vi "File_NewPathGeneartor.vi"(0 "NewPath":path, 1 "OldPath":path, 2 "NewName":string, 3 "OldName":string, 4 "NewSuffix":string, 5 "OldSuffix":string) -> (14 "PathOut":path, 16 "NameOut":string, 18 "SuffixOut":string)   [LabVIEW 2020]
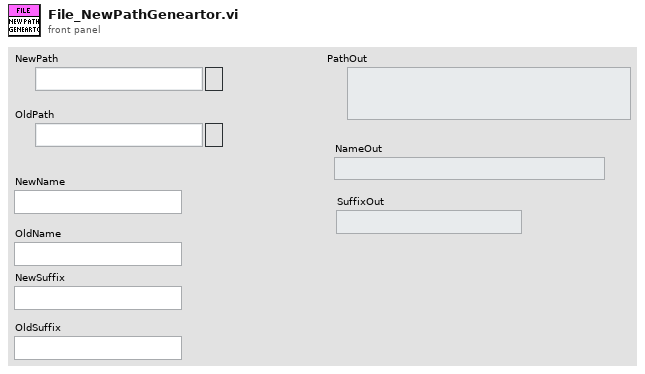
[diagram p1: front panel]
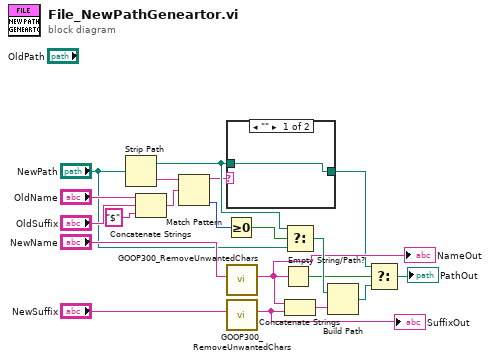
[diagram p0: block diagram]
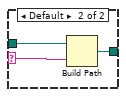
[diagram p2: hidden frame]
diagram:
  n1 = Strip Path(path="NewPath") -> (stripped path=w5:path, name=w14:string)
  n2 = Concatenate Strings("OldName", "OldSuffix", "$" ("string")) -> (w13:string)
  n3 = Match Pattern(string=w14, regular expression=w13) -> (before substring=w3:string, offset past match=w11:i32)  [unwired: 1 in, 2 out]
  n4 = Greater Or Equal To 0?(x=w11) -> (x >= 0?=w2:bool)
  n5 = case shown="\"\"" w3 {
    selector: w3 -> [_ w23]
    tunnel: w5 -> [w21 w24]
    tunnel: [w21 w22] -> w1
    frame "" {
    }
    frame Default {
      n6 = Build Path(base path=w24, name or relative path=w23) -> (appended path=w22:path)
    }
  }
  n7 = call "GOOP300_RemoveUnwantedChars.vi"("StringIn"="NewName") -> ("StringOut"=w8:string)  [unwired: 10 in]
  "NameOut" <- w8
  n8 = call "GOOP300_RemoveUnwantedChars.vi"("StringIn"="NewSuffix") -> ("StringOut"=w6:string)  [unwired: 10 in]
  "SuffixOut" <- w6
  n9 = Empty String/Path?(string/path=w8) -> (empty?=w9:bool)
  n10 = Select(t=w5, s=w2, f="NewPath") -> (s? t:f=w10:path)
  n11 = Concatenate Strings(w8, w6) -> (w7:string)
  n12 = Build Path(base path=w10, name or relative path=w7) -> (appended path=w17:path)
  n13 = Select(t=w1, s=w9, f=w17) -> (s? t:f=→"PathOut":path)
